vi "close.vi"(8 "error in (no error)":errorcluster, 11 "ScopeKeysight in":refnum<class "ScopeKeysight.lvclass">) -> (0 "error out":errorcluster)   [LabVIEW 2023, in "ScopeKeysight.lvclass"]
doc: "Close the Instrument Reference"
uses:
  ScopeKeysight.lvclass
  ScopeKeysight.lvclass/ScopeKeysight.ctl
  Scope.lvclass
  Driver/Keysight-DSQx3014T.lvlib
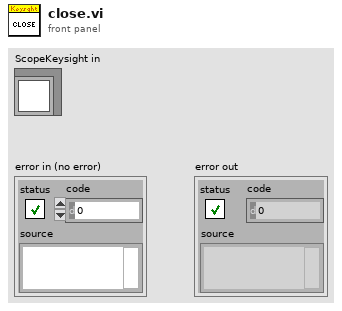
[diagram p1: front panel]
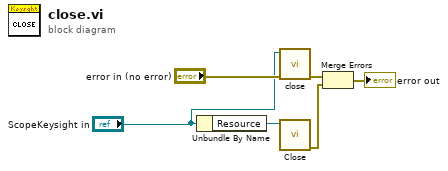
[diagram p0: block diagram]
diagram:
  n1 = Unbundle By Name("ScopeKeysight in") -> ("Resource"=w3:refnum<visa-resource-name>)
  n2 = call-parent "close.vi"("error in (no error)"="error in (no error)", "Instrument in"="ScopeKeysight in") -> ("error out"=w6:errorcluster)  [unwired: 9 in]
  n3 = call "Close.vi"("VISA resource name"=w3) -> ("error out"=w1:errorcluster)  [unwired: 10 in]
  n4 = Merge Errors(w6, w1) -> (→"error out":errorcluster)
